vi "Format Log Data.vi"(10 "Event Data String:":string="0", 11 "Event String:":string="Boiler Initialized") -> (3 "Formatted Log Data":string)   [LabVIEW 2020]
doc: "The \"Format Log Data\" subVI takes as input an Event String and Event Data String and outputs a string that is formatted properly for the Event Log File (.csv):\n\"Absolute date and time string,Event string,Event data string\n\""
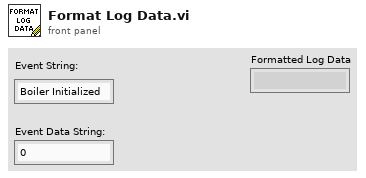
[diagram p1: front panel]
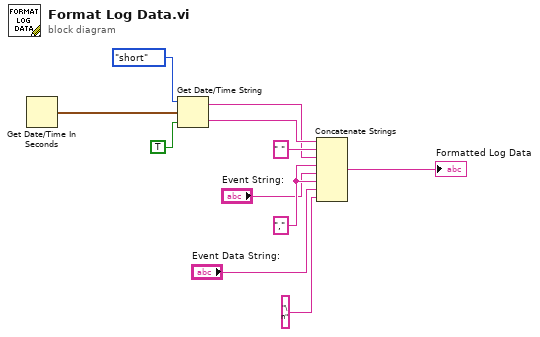
[diagram p0: block diagram]
diagram:
  w5 = "," ("string")
  n1 = Get Date/Time In Seconds() -> (seconds since 1Jan1904=w11:timestamp)
  n2 = Get Date/Time String(date format (0)=enum16{"short", "long", "abbreviated"}."short", seconds (now)=w11, want seconds? (F)=TRUE) -> (date string=w6:string, time string=w8:string)
  n3 = Concatenate Strings "Concatenate Strings"(w8, " " ("string"), w6, w5, "Event String:", w5, "Event Data String:", "\n" ("string")) -> (→"Formatted Log Data":string)
